vi "Graph Lockin vs Parameter.vi"(9 "reset?":bool, 10 "Y":dbl[](array[numeric]), 11 "X":dbl) -> (3 "Data vs Parameter":cluster{dbl[], dbl[]}[](graph))   [LabVIEW 2019, in "Transport.lvclass"]
uses:
  Transport.lvclass
  <vilib>/PRIrvin/XY Utilities/subVIs/Append (multiple).vi
  <vilib>/PRIrvin/XY Utilities/subVIs/Append (single).vi
  <vilib>/PRIrvin/XY Utilities/subVIs/Append (double array).vi
  <vilib>/PRIrvin/XY Utilities/xy_utilities.lvlib
panel:
  in  "error in (no error)":errorcluster
  out "error out":errorcluster
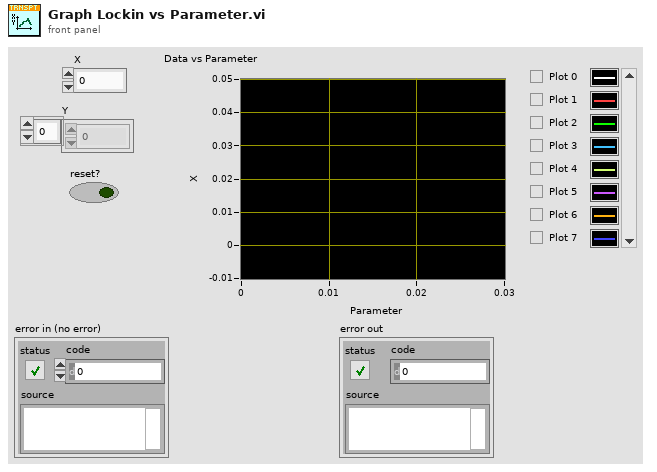
[diagram p1: front panel]
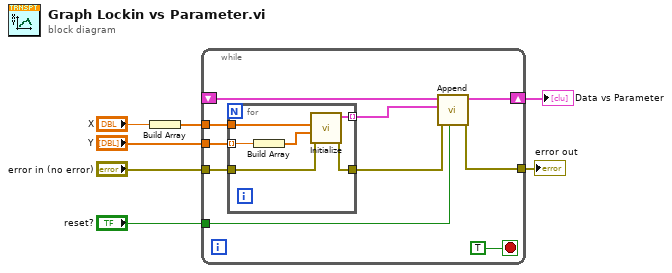
[diagram p0: block diagram]
diagram:
  n1 = Build Array("X") -> (w4:dbl[])
  n2 = while {
    tunnel: "Y" -> [w13]
    tunnel: "reset?" -> [w11]
    shift-right: [w16] -> w3
    shift-left: _ -> [w14]
    tunnel: w4 -> [w12]
    tunnel: [w9] -> w2
    tunnel: "error in (no error)" -> [w8]
    stop <- TRUE stop-if-true
    n3 = for {
      tunnel: w13 -> [w23] mode=indexing
      tunnel: [w21] -> w15 mode=indexing
      tunnel: w12 -> [w20]
      tunnel: [w19] -> w10
      tunnel: w8 -> [w18]
      n4 = Build Array(w23) -> (w22:dbl[])
      n5 = call <vilib>:"Initialize.vi"("error in (no error)"=w18, "Y-array"=w22, "X-array"=w20) -> ("error out"=w19:errorcluster, "XY-data out"=w21:cluster{"X-array":dbl[], "Y-array":dbl[]})  [unwired: 7 in]
    }
    n6 = call-poly <vilib>:"Append.vi"("Reset"=w11, "error in (no error)"=w10, "XY-data (B)"=w15, "XY-data (A)"=w14) -> ("error out"=w9:errorcluster, "XY-data out"=w16:cluster{"X-array":dbl[], "Y-array":dbl[]}[])  [unwired: 6 in]
  }
  "Data vs Parameter" <- w3
  "error out" <- w2
